vi "Test_AddSub.vi"() -> ()   [LabVIEW 2013, in "Angle.lvclass"]
uses:
  Angle.lvclass
panel:
  out "SubTestOut":dbl
  out "AddTestOut":dbl
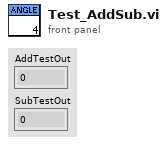
[diagram p1: front panel]
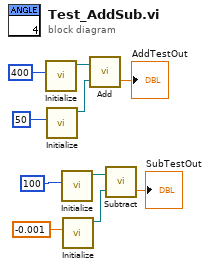
[diagram p0: block diagram]
diagram:
  n1 = call "Initialize.vi"("Input Angle (Deg.)"=400) -> ("Angle out"=w9:refnum<class "Angle.lvclass">)  [unwired: 9 in, 1 out]
  n2 = call "Initialize.vi"("Input Angle (Deg.)"=50) -> ("Angle out"=w7:refnum<class "Angle.lvclass">)  [unwired: 9 in, 1 out]
  n3 = call "Initialize.vi"("Input Angle (Deg.)"=100) -> ("Angle out"=w3:refnum<class "Angle.lvclass">)  [unwired: 9 in, 1 out]
  n4 = call "Initialize.vi"("Input Angle (Deg.)"=-0.001) -> ("Angle out"=w2:refnum<class "Angle.lvclass">)  [unwired: 9 in, 1 out]
  n5 = call "Add.vi"("AngleAdd"=w7, "Angle in"=w9) -> ("Output"=→"AddTestOut":dbl)  [unwired: 1 out]
  n6 = call "Subtract.vi"("AngleSubtract"=w2, "Angle in"=w3) -> ("Output"=→"SubTestOut":dbl)  [unwired: 1 out]
